vi "Method 1.vi"(8 "error in (no error)":errorcluster, 11 "Interface 1 in":refnum<class "Interface 1.lvclass">) -> (0 "error out":errorcluster, 3 "Interface 1 out":refnum<class "Interface 1.lvclass">)   [LabVIEW 2021, in "Interface 1.lvclass"]
uses:
  Interface 1.lvclass
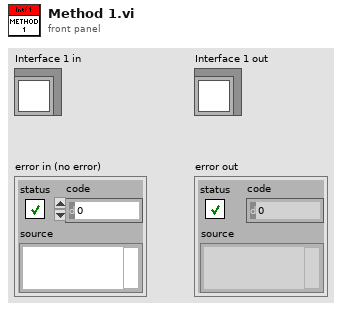
[diagram p1: front panel]
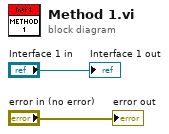
[diagram p0: block diagram]
diagram:
  "error out" <- "error in (no error)"
  "Interface 1 out" <- "Interface 1 in"
